vi "Format Rate A (GPM).vi"(3 "error out":errorcluster, 4 "Filtered Response":string, 5 "VISA resource  in":refnum<visa-resource-name>) -> (0 "error IO":errorcluster, 1 "GPM":dbl, 2 "VISA resource  out":refnum<visa-resource-name>)   [LabVIEW 2010, in "FEM-03.lvlib"]
uses:
  FEM-03.lvlib
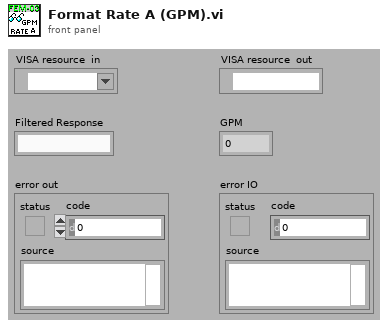
[diagram p1: front panel]
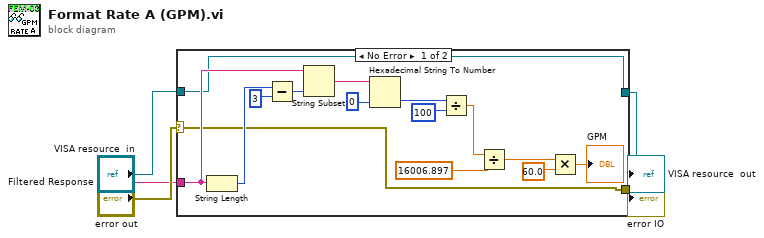
[diagram p0: block diagram]
diagram:
  n1 = case shown="No Error" "error out" {
    selector: "error out" -> [w6 w21]
    tunnel: "Filtered Response" -> [w19 _]
    tunnel: "VISA resource  in" -> [w7 w22]
    tunnel: [w7 w22] -> w5
    tunnel: [w6 w21] -> w4
    frame No Error {
      n2 = String Length(string=w19) -> (length=w18:i32)
      n3 = Subtract(x=w18, y=3) -> (x-y=w16:i32)
      n4 = String Subset(string=w19, length (rest)=w16) -> (substring=w15:string)  [unwired: 1 in]
      n5 = Hexadecimal String To Number(string=w15, default (0uL)=u32 0 ("default (0 U32)")) -> (number=w14:u32)  [unwired: 1 in, 1 out]
      n6 = Divide(x=w14, y=u32 100) -> (x/y=w8:dbl)
      n7 = Divide(x=w8, y=16006.897 ("K Factor (Pulses/GAL)")) -> (x/y=w10:dbl)
      n8 = Multiply(x=w10, y=60.0) -> (x*y=→"GPM":dbl)
    }
    frame Error {
    }
  }
  "VISA resource  out" <- w5
  "error IO" <- w4
